vi "Initialize.vi"(7 "timeout, ms (2000)":u32=2000, 8 "error in (no error)":errorcluster, 10 "port (17017)":u16=17017, 11 "address (192.168.240.181)":string="192.168.240.181") -> (0 "error out":errorcluster, 3 "SOL Camera out":refnum<class "PL SOL Instruments Camera.lvclass">)   [LabVIEW 2015, in "PL SOL Instruments Camera.lvclass"]
doc: "Initializes connection to device using specified settings."
uses:
  PL SOL Instruments Camera.lvclass
  PL SOL Instruments Camera.lvclass/PL SOL Instruments Camera.ctl
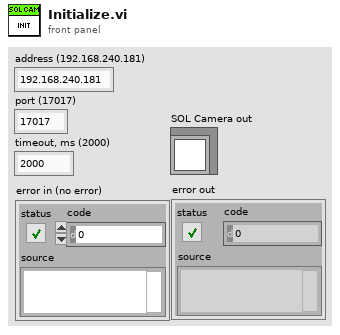
[diagram p1: front panel]
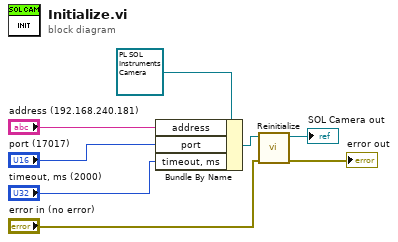
[diagram p0: block diagram]
diagram:
  n1 = Bundle By Name(cluster=refnum<class "PL SOL Instruments Camera.lvclass"> refnum ("SOL Camera out"), "address"="address (192.168.240.181)", "port"="port (17017)", "timeout, ms"="timeout, ms (2000)") -> (w5:refnum<class "PL SOL Instruments Camera.lvclass">)
  n2 = call "Reinitialize.vi"("error in (no error)"="error in (no error)", "SOL MS in"=w5) -> ("error out"=→"error out":errorcluster, "SOL Camera out"=→"SOL Camera out":refnum<class "PL SOL Instruments Camera.lvclass">)  [unwired: 8 in]
